vi "Instrument Meas EVM (LTE).vi"(6 "AutoScale (T)":bool, 7 "OPC?(T)":bool, 8 "error in":errorcluster {"code" format="%.0x"}, 10 "Timeout":u32=3000, 11 "Session In":refnum<visa-resource-name>="GPIB0::18::INSTR") -> (0 "error out":errorcluster {"code" format="%.0x"}, 1 "EVM":dbl[](array[numeric]), 2 "Data(str)":string[](array[string]), 3 "Session Out":refnum<visa-resource-name>)   [LabVIEW 2018]
doc: "Launches the Instrument I/O Assistant, which you can use to communicate with message-based instruments and graphically parse the response. For example you can communicate with an instrument that uses a serial, Ethernet, or GPIB interface."
panel:
  out "array":string[][](array[string])
  # "N Results Returned (Downlink)\nNot specified\nor n=1\nReturns comma-separated scalar results, corresponding exactly to the items returned in the Error\nSummary:\n0. EVM (%rms)\n1. String result (EVM Sym Time Adjust). NaN returned\n3. EVM Pk (%)\n2. EVM Pk Index\n3. EVM Peak Sub Car Index\n4. Data EVM (%rms) – Not available when Detection is Manual and no User is added.\n5. 3GPP-defined QPSK EVM (%rms)\n6. 3GPP-defined 16QAM EVM (%rms)\n7. 3GPP-defined 64QAM EVM (%rms)\n8. RS EVM (%rms)\n9. RS Tx. Power (dBm).\n10. OFDM Sym. Tx. Power (dBm).\n11. Freq Error (Hz)\n12. Sync Corr (%)\n13. String Result (Sync Type). NaN returned.\n14. Common Tracking Error (%rms)\n15. Symbol Clock Error (ppm)"
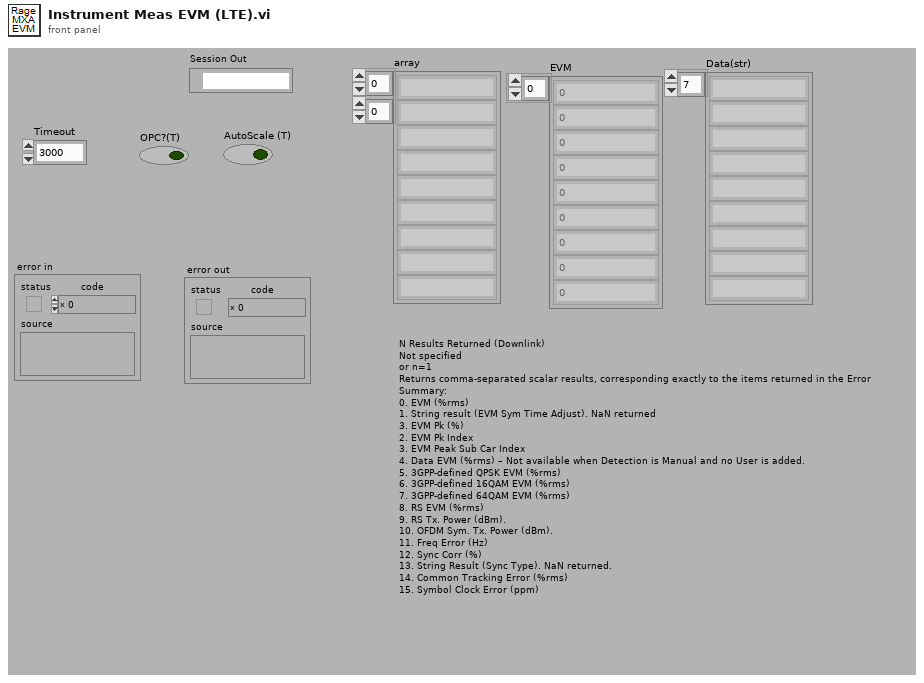
[diagram p1: front panel]
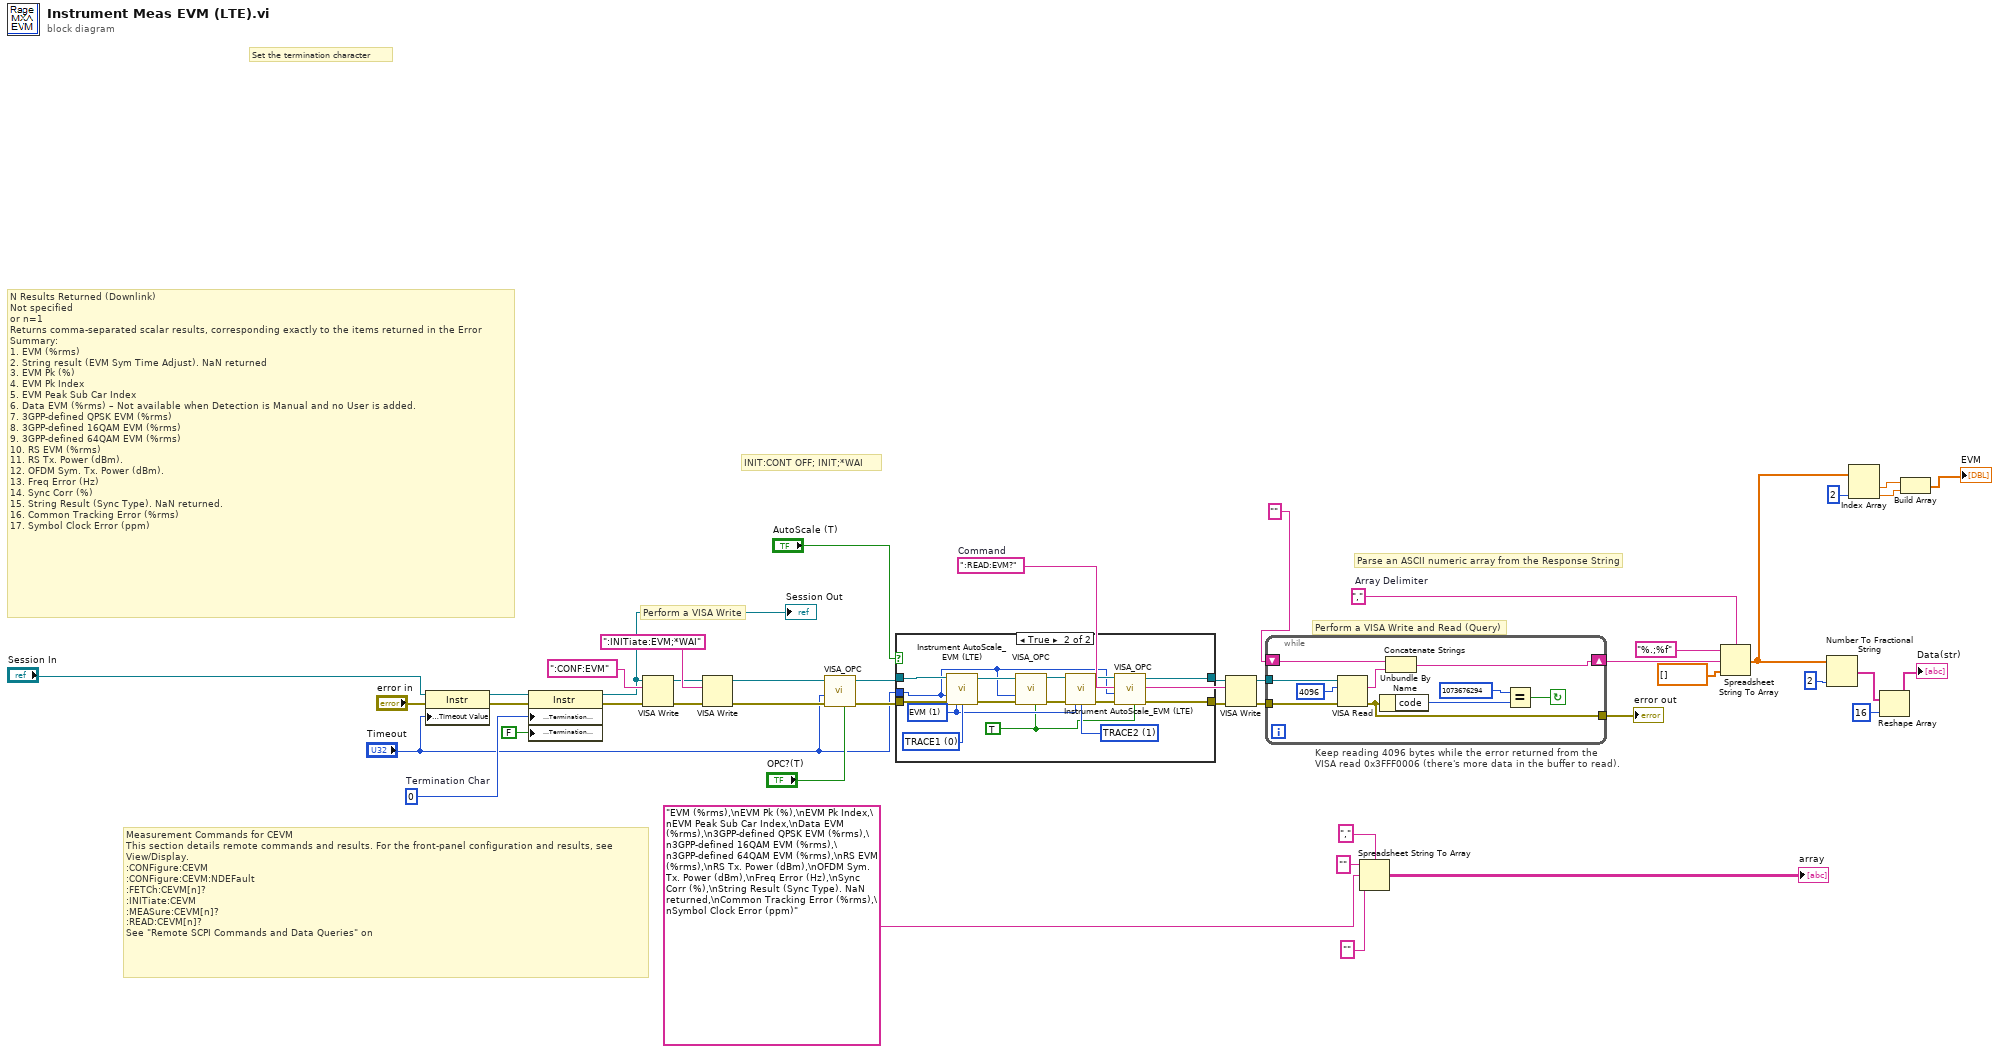
[diagram p0: block diagram]
diagram:
  w30 = ","  # Array Delimiter
  w33 = ":READ:EVM?"  # Command
  w40 = u8 0  # Termination Char
  # "INIT:CONT OFF; INIT;*WAI"
  # "Measurement Commands for CEVM\nThis section details remote commands and results. For the front-panel configuration and results, see\nView/Display.\n:CONFigure:CEVM\n:CONFigure:CEVM:NDEFault\n:FETCh:CEVM[n]?\n:INITiate:CEVM\n:MEASure:CEVM[n]?\n:READ:CEVM[n]?\nSee \"Remote SCPI Commands and Data Queries\" on"
  # "N Results Returned (Downlink)\nNot specified\nor n=1\nReturns comma-separated scalar results, corresponding exactly to the items returned in the Error\nSummary:\n1. EVM (%rms)\n2. String result (EVM Sym Time Adjust). NaN returned\n3. EVM Pk (%)\n4. EVM Pk Index\n5. EVM Peak Sub Car Index\n6. Data EVM (%rms) – Not available when Detection is Manual and no User is added.\n7. 3GPP-defined QPSK EVM (%rms)\n8. 3GPP-defined 16QAM EVM (%rms)\n9. 3GPP-defined 64QAM EVM (%rms)\n10. RS EVM (%rms)\n11. RS Tx. Power (dBm).\n12. OFDM Sym. Tx. Power (dBm).\n13. Freq Error (Hz)\n14. Sync Corr (%)\n15. String Result (Sync Type). NaN returned.\n16. Common Tracking Error (%rms)\n17. Symbol Clock Error (ppm)"
  # "Parse an ASCII numeric array from the Response String"
  # "Perform a VISA Write and Read (Query)"
  # "Keep reading 4096 bytes while the error returned from the\nVISA read 0x3FFF0006 (there's more data in the buffer to read)."
  # "Perform a VISA Write"
  # "Set the termination character"
  n1 = property class="Instr"(reference="Session In", error in="error in", "General Settings:Timeout Value"="Timeout") -> (reference out=w39:refnum<visa-resource-name>, error out=w42:errorcluster)
  n2 = property class="Instr"(reference=w39, error in=w42, "Message Based Settings:Termination Character"=w40, "Message Based Settings:Termination Character Enable"=FALSE ("enable")) -> (reference out=w25:refnum<visa-resource-name>, error out=w41:errorcluster)
  "Session Out" <- w25
  n3 = VISA Write(VISA resource name=w25, write buffer=":CONF:EVM", error in (no error)=w41) -> (VISA resource name out=w24:refnum<visa-resource-name>, error out=w27:errorcluster)  [unwired: 1 out]
  n4 = VISA Write(VISA resource name=w24, write buffer=":INITiate:EVM;*WAI" ("StaticText"), error in (no error)=w27) -> (VISA resource name out=w2:refnum<visa-resource-name>, error out=w3:errorcluster)  [unwired: 1 out]
  n5 = call "VISA_OPC.vi"("OPC(T)"="OPC?(T)", "error in"=w3, "Timeout"="Timeout", "Session In"=w2) -> ("error out"=w7:errorcluster, "Session Out"=w8:refnum<visa-resource-name>)  [unwired: 5 in, 1 out]
  n6 = case shown="True" "AutoScale (T)" {
    tunnel: w7 -> [w46 w61]
    tunnel: [w46 w51] -> w6
    tunnel: w8 -> [w45 w60]
    tunnel: [w45 w52] -> w5
    tunnel: "Timeout" -> [_ w49]
    frame False {
    }
    frame True {
      w47 = TRUE ("OPC?(T)")
      w57 = 1 items=["TRACE1", "TRACE2", "TRACE3", "TRACE4"] ("Trace")
      w59 = 0 items=["TRACE1", "TRACE2", "TRACE3", "TRACE4"] ("Trace")
      w58 = u16 1 items=["VECT", "EVM"] ("line index")
      n7 = call "Instrument AutoScale_EVM (LTE).vi"("Session In"=w60, "Timeout"=w49, "error in"=w61, "line index"=w58, "Trace"=w59) -> ("Session Out"=w56:refnum<visa-resource-name>, "error out"=w55:errorcluster)  [unwired: 9 in]
      n8 = call "VISA_OPC.vi"("OPC(T)"=w47, "error in"=w55, "Timeout"=w49, "Session In"=w56) -> ("error out"=w53:errorcluster, "Session Out"=w54:refnum<visa-resource-name>)  [unwired: 5 in, 1 out]
      n9 = call "Instrument AutoScale_EVM (LTE).vi"("Session In"=w54, "error in"=w53, "line index"=w58, "Trace"=w57) -> ("Session Out"=w50:refnum<visa-resource-name>, "error out"=w48:errorcluster)  [unwired: 10 in]
      n10 = call "VISA_OPC.vi"("OPC(T)"=w47, "error in"=w48, "Timeout"=w49, "Session In"=w50) -> ("error out"=w51:errorcluster, "Session Out"=w52:refnum<visa-resource-name>)  [unwired: 5 in, 1 out]
    }
  }
  n11 = VISA Write(VISA resource name=w5, write buffer=w33, error in (no error)=w6) -> (VISA resource name out=w36:refnum<visa-resource-name>, error out=w35:errorcluster)  [unwired: 1 out]
  n12 = while {
    tunnel: w36 -> [w68]
    shift-right: [w62] -> w29
    shift-left: "" -> [w67]
    tunnel: w35 -> [w65]
    tunnel: [w64] -> w34
    stop <- w63 continue-if-true
    n13 = VISA Read(VISA resource name=w68, byte count=u32 4096 ("byte count (0)"), error in (no error)=w65) -> (read buffer=w66:string, error out=w64:errorcluster)  [unwired: 2 out]
    n14 = Unbundle By Name(w64) -> ("code"=w70:i32)
    n15 = Concatenate Strings(w67, w66) -> (w62:string)
    n16 = Equal?(x=1073676294, y=w70) -> (x = y?=w63:bool)
  }
  "error out" <- w34
  n17 = Spreadsheet String To Array(delimiter (Tab)=",", format string="", spreadsheet string="EVM (%rms),\nEVM Pk (%),\nEVM Pk Index,\nEVM Peak Sub Car Index,\nData EVM (%rms),\n3GPP-defined QPSK EVM (%rms),\n3GPP-defined 16QAM EVM (%rms),\n3GPP-defined 64QAM EVM (%rms),\nRS EVM (%rms),\nRS Tx. Power (dBm),\nOFDM Sym. Tx. Power (dBm),\nFreq Error (Hz),\nSync Corr (%),\nString Result (Sync Type). NaN returned,\nCommon Tracking Error (%rms),\nSymbol Clock Error (ppm)", array type (2D Dbl)="" ("delimiter (Tab)")) -> (array=→"array":string[][])
  n18 = Spreadsheet String To Array(delimiter (Tab)=w30, format string="%.;%f", spreadsheet string=w29, array type (2D Dbl)=dbl[] []) -> (array=w18:dbl[])
  n19 = Number To Fractional String(number=w18, precision (6)=i16 2) -> (F-format string=w12:string[])  [unwired: 2 in]
  n20 = Index Array(array=w18, index #2=2 ("index")) -> (element #1=w17:dbl, element #2=w16:dbl)  [unwired: 1 in]
  n21 = Reshape Array(w12, 16 ("dimension size")) -> (→"Data(str)":string[])
  n22 = Build Array(w17, w16) -> (→"EVM":dbl[])
